vi "LED_spectraView.vi"() -> ()   [LabVIEW 2012]
uses:
  <vilib>/Utility/file.llb/Read From Spreadsheet File (DBL).vi
panel:
  in  "EL Intensity":string(combo)="Abs Irr"
  out "Wavelength":dbl[](array[numeric])
  out "Counts":dbl[](array[numeric])
  out "Abs Irr":dbl[](array[numeric])
  out "XY Graph":cluster{"Wavelength":dbl[], "Counts":dbl[]}(graph)
  in  "Spectrum Index":i32
  out "subarray":dbl[][](array[numeric])
  out "array":dbl[][](array[numeric])
  in  "Spectrum file":path
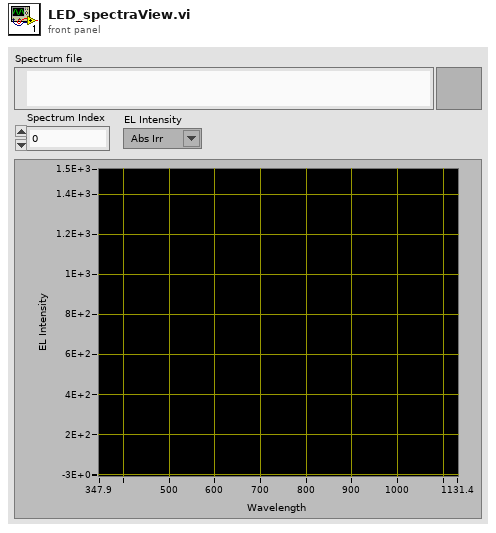
[diagram p1: front panel]
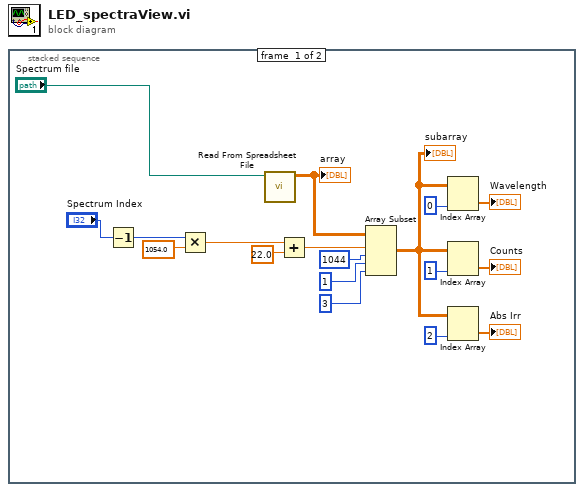
[diagram p0: block diagram]
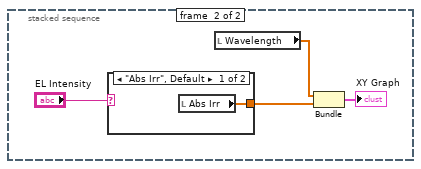
[diagram p2: hidden frame]
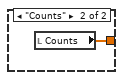
[diagram p3: hidden frame]
diagram:
  n1 = stacked-sequence {
    frame #0 {
      n2 = Decrement(x="Spectrum Index") -> (x-1=w17:i32)
      n3 = Multiply(x=w17, y=1054.0) -> (x*y=w14:dbl)
      n4 = call-poly <vilib>:"Read From Spreadsheet File.vi"("file path (dialog if empty)"="Spectrum file") -> ("all rows"=w9:dbl[][])  [unwired: 6 in, 4 out]
      "array" <- w9
      n5 = Add(x=w14, y=22.0) -> (x+y=w18:dbl)
      n6 = Array Subset(array=w9, index (row)=w18, length (row)=1044 ("length"), index (col)=1 ("index"), length (col)=3 ("length")) -> (w5:dbl[][])
      "subarray" <- w5
      n7 = Index Array(array=w5, index (col)=0 ("index")) -> (element=→"Wavelength":dbl[])  [unwired: 1 in]
      n8 = Index Array(array=w5, index (col)=1 ("length")) -> (element=→"Counts":dbl[])  [unwired: 1 in]
      n9 = Index Array(array=w5, index (col)=2 ("index")) -> (element=→"Abs Irr":dbl[])  [unwired: 1 in]
    }
    frame #1 {
      n10 = case shown="\"Abs Irr\", Default" "EL Intensity" {
        tunnel: [w23 w24] -> w19
        frame "Abs Irr", Default {
          n11 = local read "Abs Irr"() -> (w23:dbl[])
        }
        frame "Counts" {
          n12 = local read "Counts"() -> (w24:dbl[])
        }
      }
      n13 = local read "Wavelength"() -> (w21:dbl[])
      n14 = Bundle("Wavelength"=w21, "Counts"=w19) -> (→"XY Graph":cluster{"Wavelength":dbl[], "Counts":dbl[]})  [unwired: 1 in]
    }
  }
